vi "Benchmark SV Send  LV2012 - NI Verified - 1000 Byte - 1Var.vi"() -> ()   [LabVIEW 2019]
uses:
  <vilib>/Platform/TimedLoop/XDataNode/timing_clust.ctl
  <vilib>/Platform/TimedLoop/XDataNode/nitl_modes.ctl
  <vilib>/Platform/TimedLoop/XDataNode/wakeup.ctl
  <vilib>/platform/TimedLoop/XDataNode/XDataNode.xnode
  <vilib>/Platform/TimedLoop/XDataNode/XDNodeRunTimeDep.lvlib
panel:
  out "bytes written":i32
  in  "Client Closed":string="The client VI closed the connection."
  out "Time":u32
  out "Delay (ms)":u32
  out "Average Delay (ms)":dbl format="%_6f"
  out "Tries":u32
  in  "Stop":bool
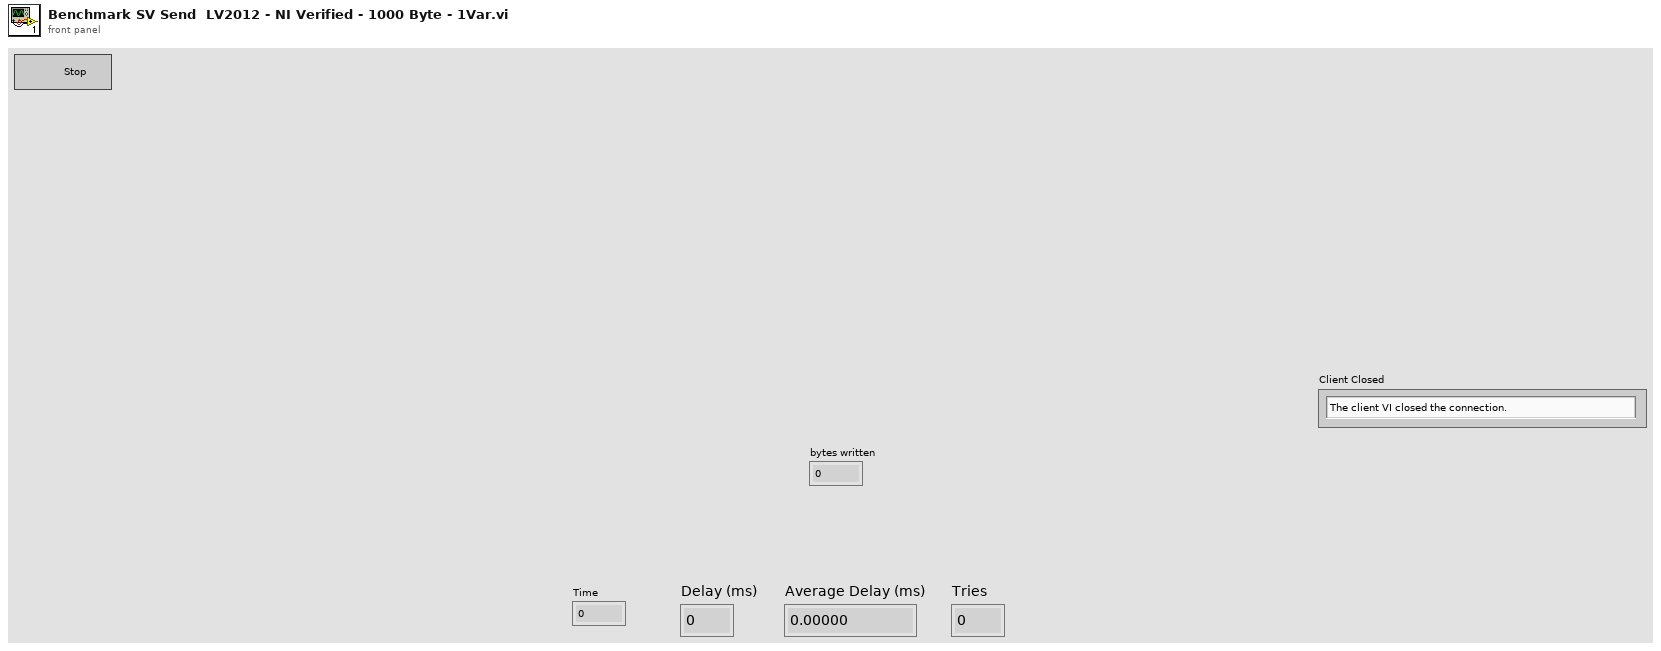
[diagram p1: front panel]
types:
  T1 = typedef "XDNodeRunTimeDep.lvlib/timing_clust.ctl" = cluster{"Expected End [f-1]":u64, "Actual End [f-1]":u64, "Finished Late? [f-1]":bool, "Expected End [i-1]":u64, "Actual End [i-1]":u64, "Finished Late? [i-1]":bool, "Expected Start [i]":u64, "Actual Start [i]":u64, "Expected Start [f]":u64, "Actual Start [f]":u64, "Source Name":string, "Structure Name":string, "Period":i64, "Deadline":i64, "Offset":i64, "Start":i64, "Priority":i32, "Timeout":i32, "Mode":T2, "Wakeup Reason":T3, "Error":errorcluster, "Source Type":string, "Secondary Source Type":string, "Global End Time":u64, "Global Start Time":u64, "Frame Duration":u64, "Iteration Duration":u64, "Assigned CPU":i32, "I/O Scan Engine Mode":u32}
  T2 = typedef "XDNodeRunTimeDep.lvlib/nitl_modes.ctl" = enum32{"No Change", "Process missed periods, maintain original phase", "Discard missed periods, maintain original phase", "Process missed periods, ignore original phase", "Discard missed periods, ignore original phase"}
  T3 = typedef "XDNodeRunTimeDep.lvlib/wakeup.ctl" = enum32{"Normal", "Aborted", "Asynchronous wakeup", "Timing source error", "Timed loop error", "Timeout"}
  T4 = cluster{i64, i64, i64, i64, i64, i64, i64, i64, i64, i64, i64, i64, i64, i64, i64, i64, i64, i64, i64, i64}
  T5 = cluster{cluster{i64, i64, i64, i64, i64, i64, i64, i64, i64, i64, i64, i64, i64, i64, i64, i64, i64, i64, i64, i64}, cluster{i64, i64, i64, i64, i64, i64, i64, i64, i64, i64, i64, i64, i64, i64, i64, i64, i64, i64, i64, i64}, cluster{i64, i64, i64, i64, i64, i64, i64, i64, i64, i64, i64, i64, i64, i64, i64, i64, i64, i64, i64, i64}, cluster{i64, i64, i64, i64, i64, i64, i64, i64, i64, i64, i64, i64, i64, i64, i64, i64, i64, i64, i64, i64}, cluster{i64, i64, i64, i64, i64, i64, i64, i64, i64, i64, i64, i64, i64, i64, i64, i64, i64, i64, i64, i64}, cluster{i64, i64, i64, i64, i64, i64, i64, i64, i64, i64, i64, i64, i64, i64, i64, i64, i64, i64, i64, i64}, cluster{i64, i64, i64, i64, i64, i64, i64, i64, i64, i64, i64, i64, i64, i64, i64, i64, i64, i64, i64, i64}, cluster{i64, i64, i64, i64, i64, i64, i64, i64, i64, i64, i64, i64, i64, i64, i64, i64, i64, i64, i64, i64}, cluster{i64, i64, i64, i64, i64, i64, i64, i64, i64, i64, i64, i64, i64, i64, i64, i64, i64, i64, i64, i64}, cluster{i64, i64, i64, i64, i64, i64, i64, i64, i64, i64, i64, i64, i64, i64, i64, i64, i64, i64, i64, i64}, cluster{i64, i64, i64, i64, i64, i64, i64, i64, i64, i64, i64, i64, i64, i64, i64, i64, i64, i64, i64, i64}, cluster{i64, i64, i64, i64, i64, i64, i64, i64, i64, i64, i64, i64, i64, i64, i64, i64, i64, i64, i64, i64}, cluster{i64, i64, i64, i64, i64, i64, i64, i64, i64, i64, i64, i64, i64, i64, i64, i64, i64, i64, i64, i64}, cluster{i64, i64, i64, i64, i64, i64, i64, i64, i64, i64, i64, i64, i64, i64, i64, i64, i64, i64, i64, i64}, cluster{i64, i64, i64, i64, i64, i64, i64, i64, i64, i64, i64, i64, i64, i64, i64, i64, i64, i64, i64, i64}, cluster{i64, i64, i64, i64, i64, i64, i64, i64, i64, i64, i64, i64, i64, i64, i64, i64, i64, i64, i64, i64}, cluster{i64, i64, i64, i64, i64, i64, i64, i64, i64, i64, i64, i64, i64, i64, i64, i64, i64, i64, i64, i64}, cluster{i64, i64, i64, i64, i64, i64, i64, i64, i64, i64, i64, i64, i64, i64, i64, i64, i64, i64, i64, i64}, cluster{i64, i64, i64, i64, i64, i64, i64, i64, i64, i64, i64, i64, i64, i64, i64, i64, i64, i64, i64, i64}, cluster{i64, i64, i64, i64, i64, i64, i64, i64, i64, i64, i64, i64, i64, i64, i64, i64, i64, i64, i64, i64}, cluster{i64, i64, i64, i64, i64, i64, i64, i64, i64, i64, i64, i64, i64, i64, i64, i64, i64, i64, i64, i64}, cluster{i64, i64, i64, i64, i64, i64, i64, i64, i64, i64, i64, i64, i64, i64, i64, i64, i64, i64, i64, i64}, cluster{i64, i64, i64, i64, i64, i64, i64, i64, i64, i64, i64, i64, i64, i64, i64, i64, i64, i64, i64, i64}, cluster{i64, i64, i64, i64, i64, i64, i64, i64, i64, i64, i64, i64, i64, i64, i64, i64, i64, i64, i64, i64}, cluster{i64, i64, i64, i64, i64, i64, i64, i64, i64, i64, i64, i64, i64, i64, i64, i64, i64, i64, i64, i64}, cluster{i64, i64, i64, i64, i64, i64, i64, i64, i64, i64, i64, i64, i64, i64, i64, i64, i64, i64, i64, i64}, cluster{i64, i64, i64, i64, i64, i64, i64, i64, i64, i64, i64, i64, i64, i64, i64, i64, i64, i64, i64, i64}, cluster{i64, i64, i64, i64, i64, i64, i64, i64, i64, i64, i64, i64, i64, i64, i64, i64, i64, i64, i64, i64}, cluster{i64, i64, i64, i64, i64, i64, i64, i64, i64, i64, i64, i64, i64, i64, i64, i64, i64, i64, i64, i64}, cluster{i64, i64, i64, i64, i64, i64, i64, i64, i64, i64, i64, i64, i64, i64, i64, i64, i64, i64, i64, i64}, cluster{i64, i64, i64, i64, i64, i64, i64, i64, i64, i64, i64, i64, i64, i64, i64, i64, i64, i64, i64, i64}, cluster{i64, i64, i64, i64, i64, i64, i64, i64, i64, i64, i64, i64, i64, i64, i64, i64, i64, i64, i64, i64}, cluster{i64, i64, i64, i64, i64, i64, i64, i64, i64, i64, i64, i64, i64, i64, i64, i64, i64, i64, i64, i64}, cluster{i64, i64, i64, i64, i64, i64, i64, i64, i64, i64, i64, i64, i64, i64, i64, i64, i64, i64, i64, i64}, cluster{i64, i64, i64, i64, i64, i64, i64, i64, i64, i64, i64, i64, i64, i64, i64, i64, i64, i64, i64, i64}, cluster{i64, i64, i64, i64, i64, i64, i64, i64, i64, i64, i64, i64, i64, i64, i64, i64, i64, i64, i64, i64}, cluster{i64, i64, i64, i64, i64, i64, i64, i64, i64, i64, i64, i64, i64, i64, i64, i64, i64, i64, i64, i64}, cluster{i64, i64, i64, i64, i64, i64, i64, i64, i64, i64, i64, i64, i64, i64, i64, i64, i64, i64, i64, i64}, cluster{i64, i64, i64, i64, i64, i64, i64, i64, i64, i64, i64, i64, i64, i64, i64, i64, i64, i64, i64, i64}, cluster{i64, i64, i64, i64, i64, i64, i64, i64, i64, i64, i64, i64, i64, i64, i64, i64, i64, i64, i64, i64}, cluster{i64, i64, i64, i64, i64, i64, i64, i64, i64, i64, i64, i64, i64, i64, i64, i64, i64, i64, i64, i64}, cluster{i64, i64, i64, i64, i64, i64, i64, i64, i64, i64, i64, i64, i64, i64, i64, i64, i64, i64, i64, i64}, cluster{i64, i64, i64, i64, i64, i64, i64, i64, i64, i64, i64, i64, i64, i64, i64, i64, i64, i64, i64, i64}, cluster{i64, i64, i64, i64, i64, i64, i64, i64, i64, i64, i64, i64, i64, i64, i64, i64, i64, i64, i64, i64}, cluster{i64, i64, i64, i64, i64, i64, i64, i64, i64, i64, i64, i64, i64, i64, i64, i64, i64, i64, i64, i64}, cluster{i64, i64, i64, i64, i64, i64, i64, i64, i64, i64, i64, i64, i64, i64, i64, i64, i64, i64, i64, i64}, cluster{i64, i64, i64, i64, i64, i64, i64, i64, i64, i64, i64, i64, i64, i64, i64, i64, i64, i64, i64, i64}, cluster{i64, i64, i64, i64, i64, i64, i64, i64, i64, i64, i64, i64, i64, i64, i64, i64, i64, i64, i64, i64}, cluster{i64, i64, i64, i64, i64, i64, i64, i64, i64, i64, i64, i64, i64, i64, i64, i64, i64, i64, i64, i64}, cluster{i64, i64, i64, i64, i64, i64, i64, i64, i64, i64, i64, i64, i64, i64, i64, i64, i64, i64, i64, i64}}
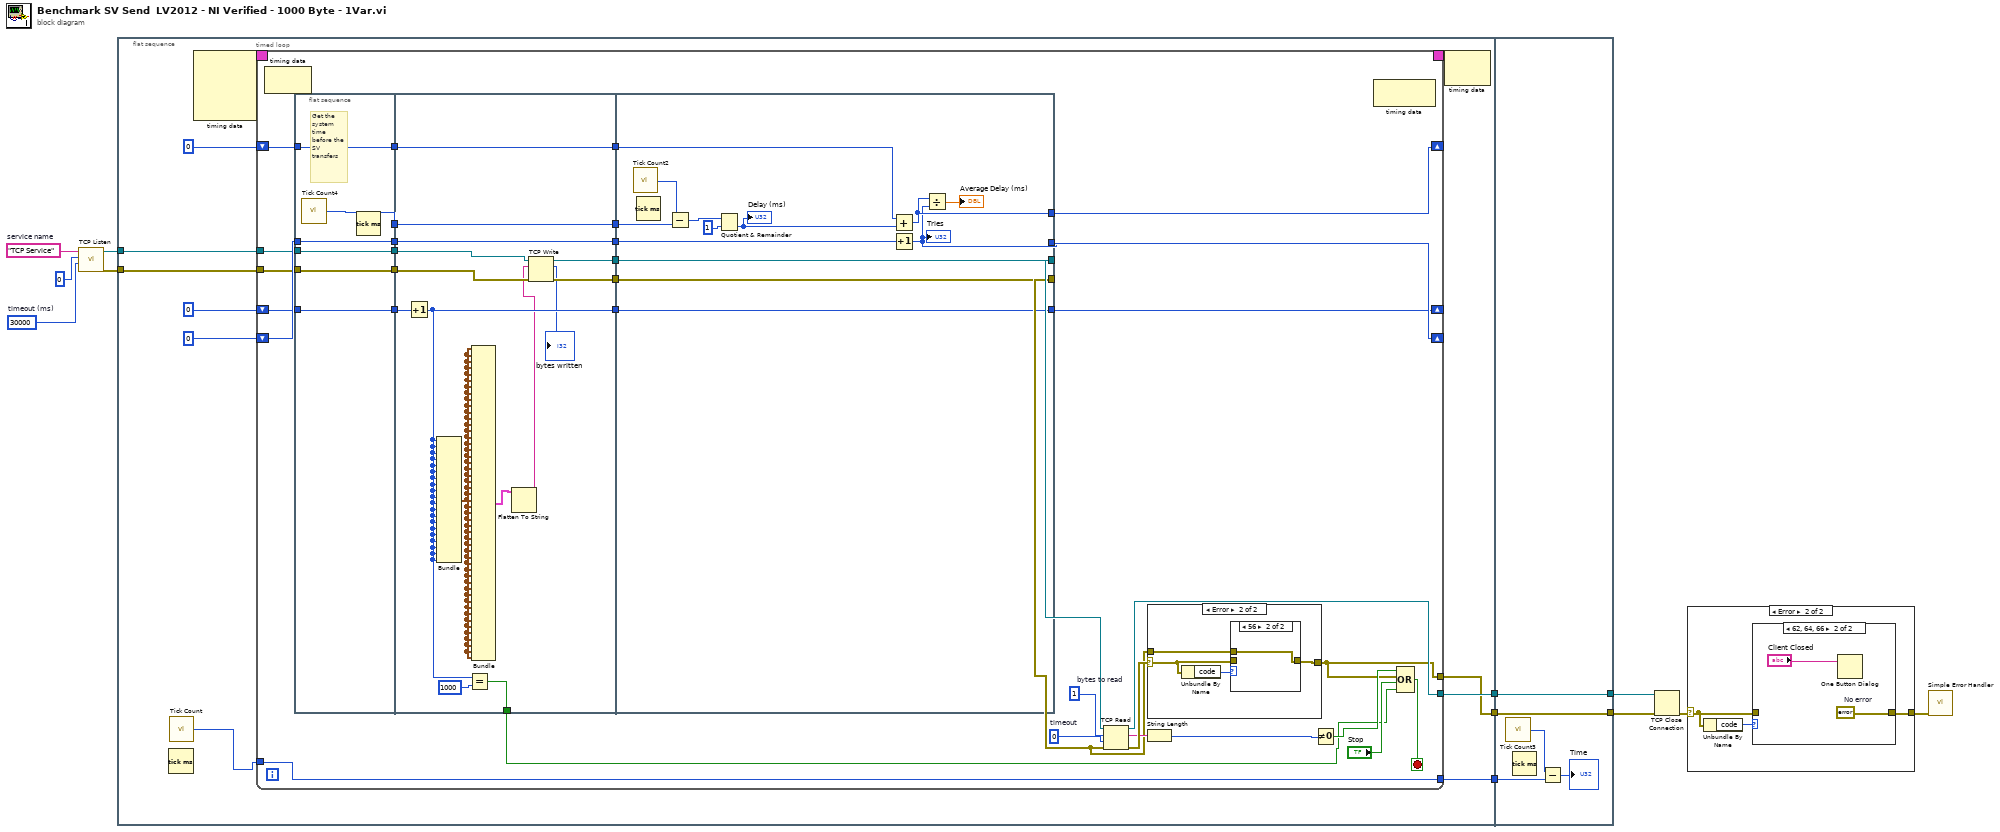
[diagram p0: block diagram]
diagram:
  w8 = "TCP Service"  # service name
  w7 = 30000  # timeout (ms)
  n1 = call <vilib>:"TCP Listen.vi"("timeout ms (wait forever: -1)"=w7, "port"=u16 0, "service name"=w8) -> ("error out"=w5:errorcluster, "connection ID"=w6:refnum<k5>)  [unwired: 4 in, 3 out]
  n2 = flat-sequence {
    tunnel: [w20] -> w12
    tunnel: w6 -> [w17]
    tunnel: w5 -> [w16]
    tunnel: [w15] -> w11
    tunnel: [w14] -> w10
    tunnel: w12 -> [w106]
    tunnel: w11 -> [w105]
    tunnel: [w105] -> w2
    tunnel: w10 -> [w104]
    tunnel: [w104] -> w1
    frame #0 {
      n3 = Tick Count (ms)() -> ()  [unwired: 1 out]
      n4 = call "Tick Count"() -> ("Tick Count(uSec)"=w13:u32)
      n5 = node-c288() -> (w19:T1)  [unwired: 4 in]
      n6 = timed-loop {
        shift-right: [w57] -> _
        shift-left: u32 0 -> [w51]
        shift-right: [w56] -> _
        shift-left: u32 0 -> [w52]
        shift-right: [w48] -> _
        shift-left: i64 0 -> [w49]
        tunnel: [w43] -> w20
        tunnel: w13 -> [w43]
        timing: w19 -> [_]
        timing-out: [_] -> w18
        tunnel: w17 -> [w41]
        tunnel: w16 -> [w39]
        tunnel: [w25] -> w15
        tunnel: [w24] -> w14
        stop <- w27 stop-if-true
        w34 = 0  # timeout
        w33 = 1  # bytes to read
        n7 = node-c288() -> ()  [unwired: 1 in, 1 out]
        n8 = flat-sequence {
          tunnel: [w67] -> w55
          tunnel: [w72] -> w54
          tunnel: [w71] -> w53
          tunnel: [w70] -> w50
          tunnel: w51 -> [w72]
          tunnel: w52 -> [w71]
          tunnel: w49 -> [w70]
          tunnel: [w69] -> w42
          tunnel: w41 -> [w69]
          tunnel: [w68] -> w40
          tunnel: w39 -> [w68]
          tunnel: [w87] -> w47
          tunnel: [w86] -> w46
          tunnel: [w85] -> w45
          tunnel: w55 -> [w87]
          tunnel: w54 -> [w86]
          tunnel: w53 -> [w85]
          tunnel: w50 -> [w84]
          tunnel: [w81] -> w44
          tunnel: [w80] -> w26
          tunnel: w42 -> [w79]
          tunnel: w40 -> [w78]
          tunnel: [w77] -> w30
          tunnel: [w76] -> w28
          tunnel: w47 -> [w100]
          tunnel: [w93] -> w57
          tunnel: w46 -> [w95]
          tunnel: [w92] -> w56
          tunnel: w45 -> [w99]
          tunnel: w44 -> [w91]
          tunnel: [w91] -> w48
          tunnel: [w90] -> w31
          tunnel: w30 -> [w90]
          tunnel: [w89] -> w29
          tunnel: w28 -> [w89]
          frame #0 {
            # "Get the system time before the SV transfers"
            n9 = call "Tick Count4"() -> ("Tick Count(uSec)"=w67:u32)
            n10 = Tick Count (ms)() -> ()  [unwired: 1 out]
          }
          frame #1 {
            n11 = Increment(x=w84) -> (x+1=w81:i64)
            n12 = Bundle(w81, w81, w81, w81, w81, w81, w81, w81, w81, w81, w81, w81, w81, w81, w81, w81, w81, w81, w81, w81) -> (w82:T4)  [unwired: 1 in]
            n13 = Equal?(x=w81, y=1000) -> (x = y?=w80:bool)
            n14 = Bundle(w82, w82, w82, w82, w82, w82, w82, w82, w82, w82, w82, w82, w82, w82, w82, w82, w82, w82, w82, w82, w82, w82, w82, w82, w82, w82, w82, w82, w82, w82, w82, w82, w82, w82, w82, w82, w82, w82, w82, w82, w82, w82, w82, w82, w82, w82, w82, w82, w82, w82) -> (w75:T5)  [unwired: 1 in]
            n15 = Flatten To String(anything=w75) -> (data string=w74:string)  [unwired: 3 in, 2 out]
            n16 = TCP Write(connection ID=w79, data in=w74, error in (no error)=w78) -> (connection ID out=w77:refnum<k5>, bytes written=→"bytes written":i32, error out=w76:errorcluster)  [unwired: 1 out]
          }
          frame #2 {
            n17 = call "Tick Count2"() -> ("Tick Count(uSec)"=w88:u32)
            n18 = Tick Count (ms)() -> ()  [unwired: 1 out]
            n19 = Subtract(x=w88, y=w100) -> (x-y=w98:u32)
            n20 = Quotient & Remainder(x=w98, y=u32 1) -> (floor(x/y)=w96:u32)  [unwired: 1 out]
            "Delay (ms)" <- w96
            n21 = Add(x=w95, y=w96) -> (x+y=w93:u32)
            n22 = Increment(x=w99) -> (x+1=w92:u32)
            "Tries" <- w92
            n23 = Divide(x=w93, y=w92) -> (x/y=→"Average Delay (ms)":dbl)
          }
        }
        n24 = TCP Read(connection ID=w31, bytes to read=w33, error in (no error)=w29, 9:w34) -> (connection ID out=w25:refnum<k5>, data out=w36:string, error out=w38:errorcluster)  [unwired: 1 out]
        n25 = case shown="Error" w38 {
          selector: w38 -> [w58 w61]
          tunnel: [w58 w59] -> w24
          tunnel: w29 -> [_ w60]
          frame No Error {
          }
          frame Error {
            n26 = Unbundle By Name(w61) -> ("code"=w62:i32)
            n27 = case shown="56" w62 {
              tunnel: w61 -> [w63 _]
              tunnel: w60 -> [_ w64]
              tunnel: [w63 w64] -> w59
              frame Default {
              }
              frame 56 {
              }
            }
          }
        }
        n28 = String Length(string=w36) -> (length=w35:i32)
        n29 = Not Equal To 0?(x=w35) -> (x != 0?=w37:bool)
        n30 = node-c288() -> ()  [unwired: 1 in, 1 out]
        n31 = Compound Arithmetic op=OR(w37, w24, "Stop", w26) -> (w27:bool)
      }
      n32 = node-c288(w18) -> ()  [unwired: 1 out]
    }
    frame #1 {
      n33 = call "Tick Count3"() -> ("Tick Count(uSec)"=w103:u32)
      n34 = Tick Count (ms)() -> ()  [unwired: 1 out]
      n35 = Subtract(x=w103, y=w106) -> (x-y=→"Time":u32)
    }
  }
  n36 = TCP Close Connection(connection ID=w2, error in (no error)=w1) -> (error out=w4:errorcluster)  [unwired: 2 out]
  n37 = case shown="Error" w4 {
    selector: w4 -> [w108 w110]
    tunnel: [w108 w109] -> w3
    frame No Error {
    }
    frame Error {
      n38 = Unbundle By Name(w110) -> ("code"=w111:i32)
      n39 = case shown="62, 64, 66" w111 {
        tunnel: w110 -> [w112 _]
        tunnel: [w112 w114] -> w109
        frame Default {
        }
        frame 62, 64, 66 {
          w114 = errorcluster {"status"=FALSE, "code"=0, "source"=""}  # No error
          n40 = One Button Dialog(message="Client Closed") -> ()  [unwired: 1 in, 1 out]
        }
      }
    }
  }
  n41 = call <vilib>:"Simple Error Handler.vi"("error in (no error)"=w3) -> ()  [unwired: 1 in, 8 out]
